vi "Simple Web Server.vi"() -> ()   [LabVIEW 2014]
uses:
  <vilib>/LabVIEW Universal Transcriptor/ESP8266 WiFi Wrapper/ESP8266 WiFi Wrapper.lvlib
panel:
  in  "DNS address":u8[](array[numeric])=[1, 2, 3, 4]
  in  "IP address":u8[](array[numeric])=[192, 168, 0, 42]
  in  "Gateway":u8[](array[numeric])=[192, 168, 0, 1]
  in  "Subnet mask":u8[](array[numeric])=[255, 255, 255, 0]
  in  "SSID":string="ESP8266 Wifi Example"
  in  "Listen Port":u8=80
  in  "error in (no error)":errorcluster
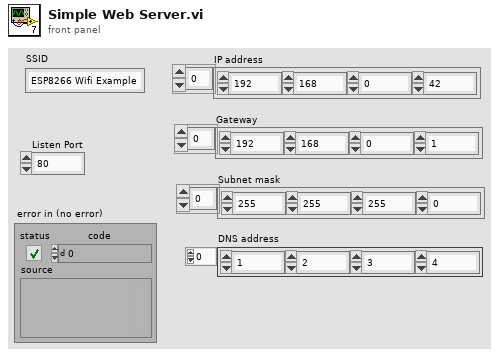
[diagram p1: front panel]
types:
  T1 = enum16{"WIFI_OFF", "WIFI_STA", "WIFI_AP", "WIFI_AP_STA"}
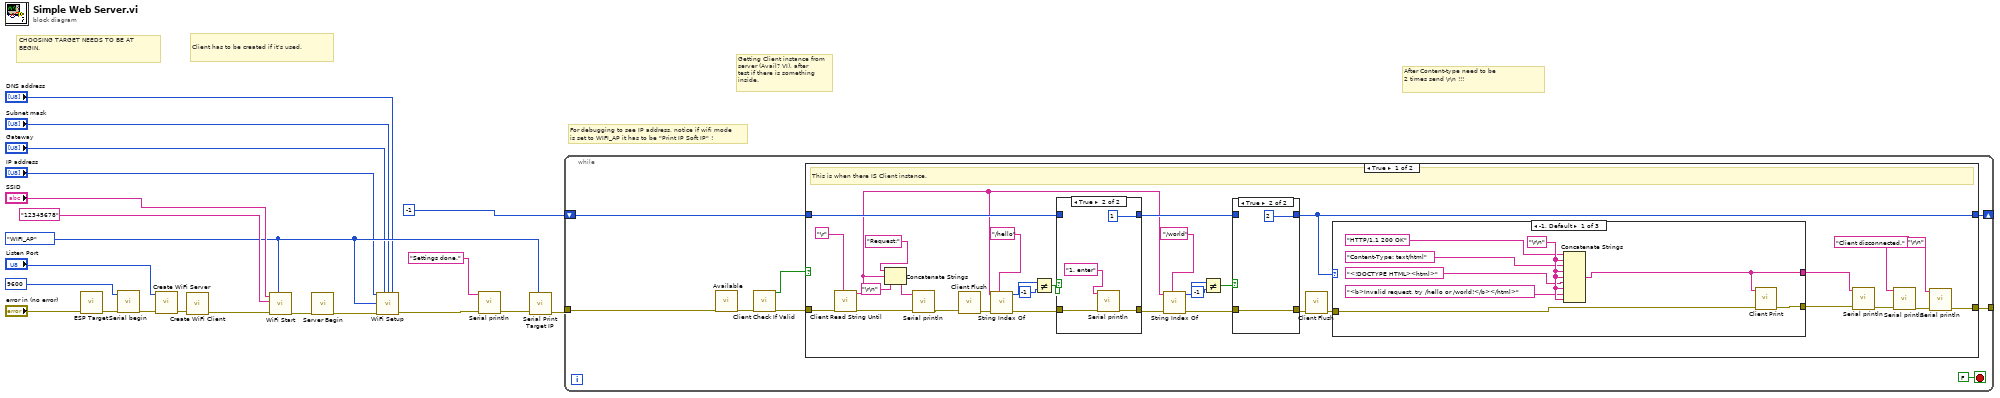
[diagram p0: block diagram]
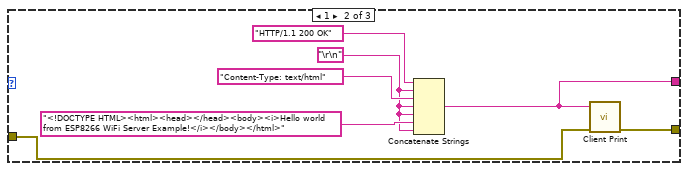
[diagram p2: hidden frame]
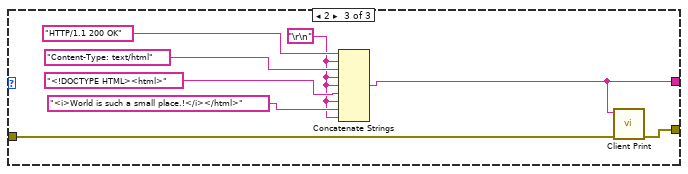
[diagram p3: hidden frame]
diagram:
  w5 = T1."WIFI_AP" ("WiFi Server Mode")
  # "For debugging to see IP address, notice if wifi mode\nis set to WIFI_AP it has to be \"Print IP Soft IP\" !"
  # "After Content-type need to be\n2 times send \\r\\n !!!"
  # "Getting Client instance from\nserver (Avail? VI), after\ntest if there is something\ninside."
  # "CHOOSING TARGET NEEDS TO BE AT BEGIN."
  # "Client has to be created if it's used."
  n1 = call <vilib>:"ESP Target.vi"("Error In"="error in (no error)") -> ("Error Out"=w13:errorcluster)  [unwired: 10 in]
  n2 = call "Serial begin.vi"("Error In"=w13, "speed (Bd)"=u32 9600 ("Speed")) -> ("Error Out"=w12:errorcluster)  [unwired: 9 in]
  n3 = call <vilib>:"Create WiFi Server.vi"("Error In"=w12, "Listen Port"="Listen Port") -> ("Error Out"=w19:errorcluster)  [unwired: 9 in]
  n4 = call <vilib>:"Create WiFi Client.vi"("Error In"=w19) -> ("Error Out"=w17:errorcluster)  [unwired: 10 in]
  n5 = call <vilib>:"WiFi Start.vi"("WiFi Mode"=w5, "Error In"=w17, "Password"="12345678", "SSID"="SSID") -> ("Error Out"=w8:errorcluster)  [unwired: 7 in]
  n6 = call <vilib>:"Server Begin.vi"("Error In"=w8) -> ("Error Out"=w6:errorcluster)  [unwired: 10 in]
  n7 = call <vilib>:"WiFi Setup.vi"("IP address"="IP address", "Gateway address"="Gateway", "Subnet mask"="Subnet mask", "DNS address"="DNS address", "WiFi Mode"=w5, "Error In"=w6) -> ("Error Out"=w7:errorcluster)  [unwired: 9 in]
  n8 = call "Serial println.vi"("Error In"=w7, "string in"="Settings done." ("String")) -> ("Error Out"=w9:errorcluster)  [unwired: 9 in]
  n9 = call <vilib>:"Serial Print Target IP.vi"("WiFi Mode"=w5, "Error In"=w9) -> ("Error Out"=w14:errorcluster)  [unwired: 9 in]
  n10 = while {
    tunnel: [w27] -> _
    shift-right: [w25] -> _
    shift-left: i8 -1 -> [w26]
    tunnel: w14 -> [w23]
    stop <- FALSE stop-if-true
    n11 = call <vilib>:"Available.vi"("Error In"=w23) -> ("Error Out"=w22:errorcluster)  [unwired: 10 in]
    n12 = call <vilib>:"Client Check If Valid.vi"("Error In"=w22) -> ("Error Out"=w24:errorcluster, "Is Null?"=w28:bool)  [unwired: 9 in]
    n13 = case shown="True" w28 {
      tunnel: w24 -> [w61 w96]
      tunnel: [w33 w96] -> w27
      tunnel: [w45 w95] -> w25
      tunnel: w26 -> [w48 w95]
      frame True {
        # "This is when there IS Client instance."
        n14 = call <vilib>:"Client Read String Until.vi"("Terminator char"="\r" ("Carriage Return Constant"), "Error In"=w61) -> ("Error Out"=w40:errorcluster, "Read String"=w42:string)  [unwired: 8 in]
        n15 = Concatenate Strings("Request:" ("string"), w42, "\r\n" ("End of Line Constant")) -> (w38:string)
        n16 = call "Serial println.vi"("Error In"=w40, "string in"=w38) -> ("Error Out"=w39:errorcluster)  [unwired: 9 in]
        n17 = call <vilib>:"Client Flush.vi"("Error In"=w39) -> ("Error Out"=w60:errorcluster)  [unwired: 10 in]
        n18 = call <vilib>:"String Index Of.vi"("IndexOf String"="/hello", "Error In"=w60, "Input String"=w42) -> ("Error Out"=w55:errorcluster, "index"=w58:i8)  [unwired: 7 in]
        n19 = Not Equal?(x=w58, y=i8 -1) -> (x != y?=w57:bool)
        n20 = case shown="True" w57 {
          tunnel: [w90 w93] -> w49
          tunnel: w55 -> [w90 w92]
          tunnel: [w89 i8 1] -> w47
          tunnel: w48 -> [w89 _]
          frame False {
          }
          frame True {
            n21 = call "Serial println.vi"("Error In"=w92, "string in"="1. enter" ("String")) -> ("Error Out"=w93:errorcluster)  [unwired: 9 in]
          }
        }
        n22 = call <vilib>:"String Index Of.vi"("IndexOf String"="/world", "Error In"=w49, "Input String"=w42) -> ("Error Out"=w54:errorcluster, "index"=w51:i8)  [unwired: 7 in]
        n23 = Not Equal?(x=w51, y=i8 -1) -> (x != y?=w52:bool)
        n24 = case shown="True" w52 {
          tunnel: [w86 w88] -> w46
          tunnel: w54 -> [w86 w88]
          tunnel: [w85 i8 2] -> w45
          tunnel: w47 -> [w85 _]
          frame False {
          }
          frame True {
          }
        }
        n25 = call <vilib>:"Client Flush.vi"("Error In"=w46) -> ("Error Out"=w44:errorcluster)  [unwired: 10 in]
        n26 = case shown="-1, Default" w45 {
          tunnel: [w68 w76 w83] -> w37
          tunnel: w44 -> [w69 w72 w84]
          tunnel: [w62 w71 w77] -> w36
          frame -1, Default {
            w67 = "\r\n" ("End of Line Constant")
            n27 = Concatenate Strings("HTTP/1.1 200 OK", w67, "Content-Type: text/html", w67, w67, "<!DOCTYPE HTML><html>", w67, "<b>Invalid request, try /hello or /world!</b></html>", w67) -> (w62:string)
            n28 = call <vilib>:"Client Print.vi"("Error In"=w69, "Input String"=w62) -> ("Error Out"=w68:errorcluster)  [unwired: 9 in]
          }
          frame 1 {
            w70 = "\r\n" ("End of Line Constant")
            n29 = Concatenate Strings("HTTP/1.1 200 OK", w70, "Content-Type: text/html", w70, w70, "<!DOCTYPE HTML><html><head></head><body><i>Hello world from ESP8266 WiFi Server Example!</i></body></html>", w70) -> (w71:string)
            n30 = call <vilib>:"Client Print.vi"("Error In"=w72, "Input String"=w71) -> ("Error Out"=w76:errorcluster)  [unwired: 9 in]
          }
          frame 2 {
            w78 = "\r\n" ("End of Line Constant")
            n31 = Concatenate Strings("HTTP/1.1 200 OK", w78, "Content-Type: text/html", w78, w78, "<!DOCTYPE HTML><html>", w78, "<i>World is such a small place.!</i></html>", w78) -> (w77:string)
            n32 = call <vilib>:"Client Print.vi"("Error In"=w84, "Input String"=w77) -> ("Error Out"=w83:errorcluster)  [unwired: 9 in]
          }
        }
        n33 = call "Serial println.vi"("Error In"=w37, "string in"=w36) -> ("Error Out"=w35:errorcluster)  [unwired: 9 in]
        n34 = call "Serial println.vi"("Error In"=w35, "string in"="Client disconnected." ("String")) -> ("Error Out"=w34:errorcluster)  [unwired: 9 in]
        n35 = call "Serial println.vi"("Error In"=w34, "string in"="\r\n" ("End of Line Constant")) -> ("Error Out"=w33:errorcluster)  [unwired: 9 in]
      }
      frame False {
        # "No Client instance, do nothing."
      }
    }
  }
